vi "Read Highlighted Rows.vi"(8 "error in (no error)":errorcluster, 11 "Array MCListbox Refnum":refnum<vi>) -> (0 "error out":errorcluster, 1 "Row Indices":i32[](array[numeric]), 2 "Item Names":string[][](array[string]))   [LabVIEW 2020, in "ListboxExtensions.lvlib"]
doc: "读取高亮显示的行"
uses:
  ListboxExtensions.lvlib
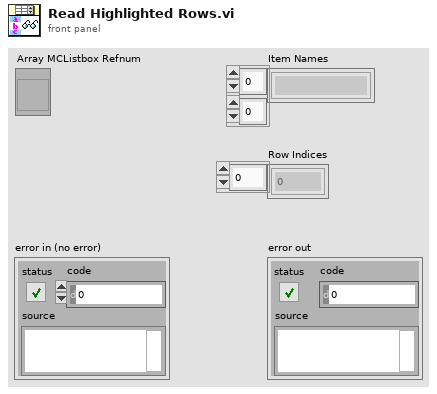
[diagram p1: front panel]
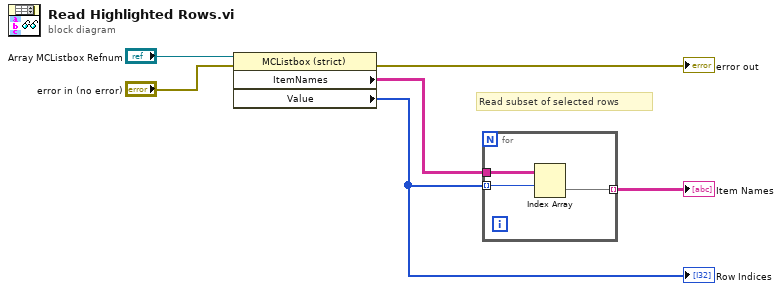
[diagram p0: block diagram]
diagram:
  # "Read subset of selected rows"
  n1 = property class="MCListbox (strict)"(reference="Array MCListbox Refnum", error in="error in (no error)") -> (error out=→"error out":errorcluster, "ItemNames"=w3:string[][], "Value"=w4:i32[])  [unwired: 1 out]
  "Row Indices" <- w4
  n2 = for {
    tunnel: [w9] -> w5 mode=indexing
    tunnel: w4 -> [w8] mode=indexing
    tunnel: w3 -> [w7]
    n3 = Index Array(array=w7, index (row)=w8) -> (element=w9:string[])  [unwired: 1 in]
  }
  "Item Names" <- w5
